vi "Disable Diagram.vi"() -> ()   [LabVIEW 2019]
panel:
  out "Result":bool
  in  "Numeric 2":dbl
  in  "Numeric":dbl
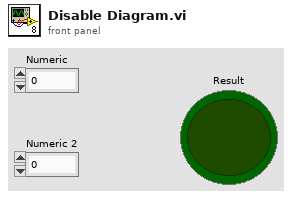
[diagram p1: front panel]
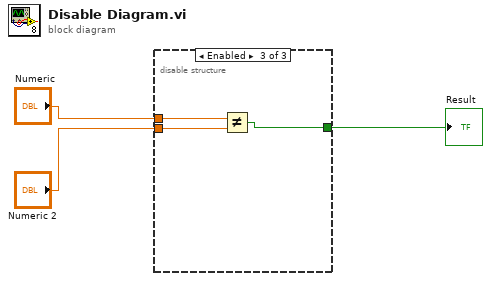
[diagram p0: block diagram]
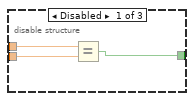
[diagram p2: hidden frame]
diagram:
  n1 = disable-structure shown="Enabled" {
    disable-tunnel: "Numeric" -> [w6 _ w9]
    disable-tunnel: "Numeric 2" -> [w5 _ w8]
    disable-tunnel: [w4 _ w7] -> w1
    frame Disabled {
      n2 = Equal?(x=w6, y=w5) -> (x = y?=w4:bool)
    }
    frame Disabled {
    }
    frame Enabled {
      n3 = Not Equal?(x=w9, y=w8) -> (x != y?=w7:bool)
    }
  }
  "Result" <- w1
